vi "Crossing Balls.vi"() -> ()   [LabVIEW 2023]
uses:
  Crossing Balls.ctl
  <vilib>/numeric/Random Number (Range) U64.vi
  <vilib>/numeric/sub_Random U32.vi
panel:
  out "Combinations":i32
  out "2D Picture":picture
  in  "stop":bool
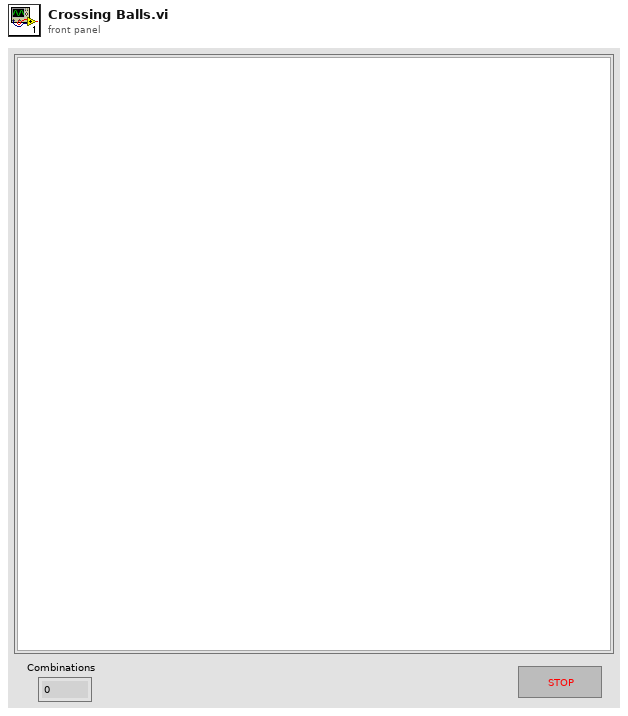
[diagram p1: front panel]
types:
  T1 = typedef "Crossing Balls.ctl" = enum16{"initialize", "InRange", "DrawPicture"}
  T2 = cluster{"horizontal":enum16{"left", "center", "right"}, "vertical":enum16{"top", "center", "bottom"}}
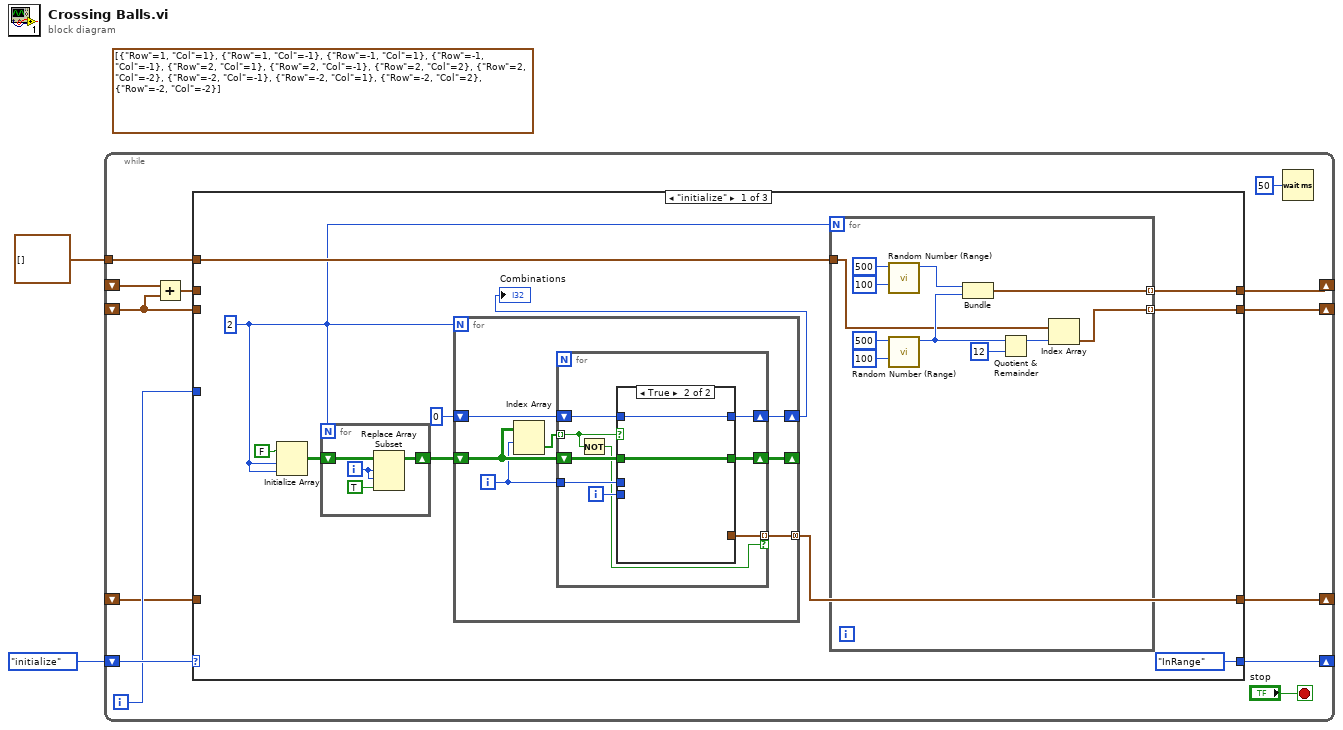
[diagram p0: block diagram]
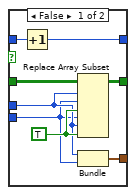
[diagram p2: hidden frame]
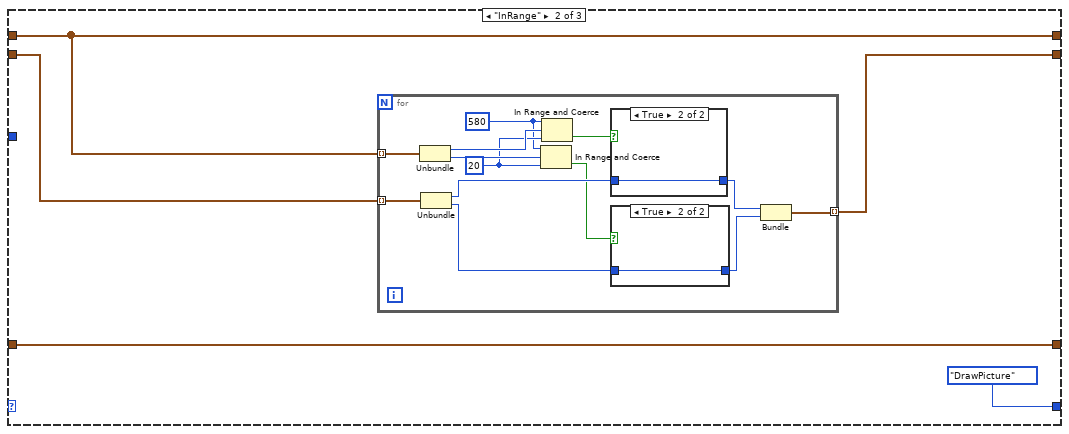
[diagram p3: hidden frame]
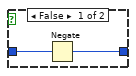
[diagram p4: hidden frame]
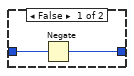
[diagram p5: hidden frame]
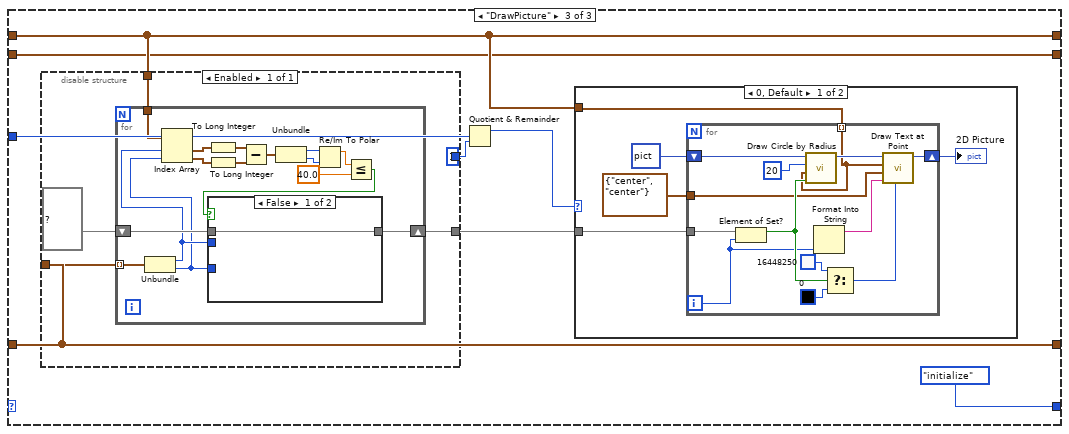
[diagram p6: hidden frame]
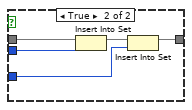
[diagram p7: hidden frame]
diagram:
  (unwired) cluster{"Row":i32, "Col":i32}[] [{"Row"=1, "Col"=1}, {"Row"=1, "Col"=-1}, {"Row"=-1, "Col"=1}, {"Row"=-1, "Col"=-1}, {"Row"=2, "Col"=1}, {"Row"=2, "Col"=-1}, {"Row"=2, "Col"=2}, {"Row"=2, "Col"=-2}, {"Row"=-2, "Col"=-1}, {"Row"=-2, "Col"=1}, {"Row"=-2, "Col"=2}, {"Row"=-2, "Col"=-2}]
  n1 = while {
    shift-right: [w12] -> _
    shift-left: Crossing_Balls."initialize" -> [w13]
    tunnel: cluster{i32, i32}[] [] -> [w10]
    shift-right: [w8] -> _
    shift-left: _ -> [w5]
    shift-right: [w9] -> _
    shift-left: _ -> [w7]
    shift-right: [w4] -> _
    shift-left: _ -> [w3]
    i -> [w11]
    stop <- "stop" stop-if-true
    n2 = Add(x=w7, y=w5) -> (x+y=w6:cluster{u64, u64}[])
    n3 = case shown="\"initialize\"" w13 {
      tunnel: w10 -> [w26 _ _]
      tunnel: [Crossing_Balls."InRange" enum16{"initialize", "InRange", "DrawPicture"}."DrawPicture" Crossing_Balls."initialize"] -> w12
      tunnel: w11 -> [_ _ w99]
      tunnel: [w25 w71 w96] -> w9
      tunnel: [w24 w69 w94] -> w8
      tunnel: w6 -> [_ w71 w96]
      tunnel: w5 -> [_ w70 w94]
      tunnel: [w17 w68 w93] -> w4
      tunnel: w3 -> [_ w68 w93]
      frame "initialize" {
        w16 = 2
        n4 = Initialize Array(FALSE, w16, w16) -> (w21:bool[][])
        n5 = for {
          N: w16 -> [_]
          shift-right: [w53] -> w20
          shift-left: w21 -> [w56]
          i -> [w55]
          n6 = Replace Array Subset(array=w56, new element=TRUE ("new element/subarray"), index (row)=w55, index (col)=w55) -> (w53:bool[][])
        }
        n7 = for {
          N: w16 -> [_]
          shift-right: [w28] -> _
          shift-left: w20 -> [w33]
          shift-right: [w29] -> w18
          shift-left: 0 -> [w30]
          tunnel: [w27] -> w17 mode=concatenating
          i -> [w31]
          n8 = Index Array(array=w33, index (row)=w31) -> (element=w32:bool[])  [unwired: 1 in]
          n9 = for {
            shift-right: [w39] -> w28
            shift-left: w33 -> [w42]
            tunnel: w32 -> [w36] mode=indexing
            tunnel: w31 -> [w41]
            shift-right: [w37] -> w29
            shift-left: w30 -> [w38]
            tunnel: [w35] -> w27 mode=indexing if=w34
            i -> [w40]
            n10 = Not(x=w36) -> (.not. x?=w34:bool)
            n11 = case shown="True" w36 {
              tunnel: w42 -> [w50 w51]
              tunnel: w41 -> [w45 _]
              tunnel: w40 -> [w44 _]
              tunnel: [w49 w51] -> w39
              tunnel: w38 -> [w47 w52]
              tunnel: [w46 w52] -> w37
              tunnel: [w43 _] -> w35
              frame False {
                w48 = TRUE
                n12 = Increment(x=w47) -> (x+1=w46:i32)
                n13 = Replace Array Subset(array=w50, new element #1=w48, index (row) #1=w45, index (col) #1=w44, new element #2=w48, index (row) #2=w44, index (col) #2=w45) -> (w49:bool[][])
                n14 = Bundle(w45, w44) -> (w43:cluster{i32, i32})  [unwired: 1 in]
              }
              frame True {
              }
            }
          }
        }
        "Combinations" <- w18
        n15 = for {
          N: w16 -> [_]
          tunnel: [w59] -> w25 mode=indexing
          tunnel: [w58] -> w24 mode=indexing
          tunnel: w26 -> [w57]
          n16 = call-poly <vilib>:"Random Number (Range).vi"("lower bound (0)"=u64 100, "upper bound (100)"=u64 500) -> ("number"=w63:u64)  [unwired: 9 in]
          n17 = call-poly <vilib>:"Random Number (Range).vi"("lower bound (0)"=u64 100, "upper bound (100)"=u64 500) -> ("number"=w62:u64)  [unwired: 9 in]
          n18 = Bundle("number"=w63, "number"=w62) -> (w59:cluster{"number":u64, "number":u64})  [unwired: 1 in]
          n19 = Quotient & Remainder(x=w62, y=u64 12) -> (x-y*floor(x/y)=w60:u64)  [unwired: 1 out]
          n20 = Index Array(array=w57, index=w60) -> (element=w58:cluster{i32, i32})
        }
      }
      frame "InRange" {
        n21 = for {
          tunnel: w71 -> [w85] mode=indexing
          tunnel: w70 -> [w84] mode=indexing
          tunnel: [w73] -> w69 mode=indexing
          w75 = u64 20 ("lower limit")
          w74 = u64 580 ("upper limit")
          n22 = Unbundle(w85) -> (w82:u64, w83:u64)
          n23 = Unbundle(w84) -> (w81:i32, w79:i32)
          n24 = In Range and Coerce(upper limit=w74, x=w83, lower limit=w75) -> (In Range?=w76:bool)  [unwired: 1 out]
          n25 = In Range and Coerce(upper limit=w74, x=w82, lower limit=w75) -> (In Range?=w77:bool)  [unwired: 1 out]
          n26 = case shown="True" w77 {
            tunnel: w81 -> [w90 w91]
            tunnel: [w89 w91] -> w80
            frame False {
              n27 = Negate(x=w90) -> (-x=w89:i32)
            }
            frame True {
            }
          }
          n28 = case shown="True" w76 {
            tunnel: w79 -> [w87 w88]
            tunnel: [w86 w88] -> w78
            frame False {
              n29 = Negate(x=w87) -> (-x=w86:i32)
            }
            frame True {
            }
          }
          n30 = Bundle(w80, w78) -> (w73:cluster{i32, i32})  [unwired: 1 in]
        }
      }
      frame "DrawPicture" {
        n31 = disable-structure shown="Enabled" {
          disable-tunnel: [w103] -> w98
          disable-tunnel: w96 -> [w102]
          disable-tunnel: w93 -> [w101]
          disable-tunnel: [1 ("y")] -> w92
          frame Enabled {
            n32 = for {
              shift-right: [w109] -> w103
              shift-left: set{i32} {} ("set") -> [w110]
              tunnel: w102 -> [w120]
              tunnel: w101 -> [w107] mode=indexing
              n33 = Unbundle(w107) -> (w106:i32, w105:i32)
              n34 = Index Array(array=w120, index #1=w106, index #2=w105) -> (element #1=w119:cluster{u64, u64}, element #2=w118:cluster{u64, u64})
              n35 = To Long Integer(number=w119) -> (32bit integer=w116:cluster{i32, i32})
              n36 = To Long Integer(number=w118) -> (32bit integer=w117:cluster{i32, i32})
              n37 = Subtract(x=w116, y=w117) -> (x-y=w115:cluster{i32, i32})
              n38 = Unbundle(w115) -> (w114:i32, w113:i32)
              n39 = Re/Im To Polar(2:w113, 3:w114) -> (1:w112:dbl)  [unwired: 1 out]
              n40 = Less Or Equal?(x=w112, y=40.0) -> (x <= y?=w108:bool)
              n41 = case shown="False" w108 {
                tunnel: w110 -> [w121 w126]
                tunnel: [w121 w124] -> w109
                tunnel: w106 -> [_ w123]
                tunnel: w105 -> [_ w122]
                frame False {
                }
                frame True {
                  n42 = Insert Into Set(10:w123, 11:w126) -> (3:w125:set{i32})  [unwired: 1 out]
                  n43 = Insert Into Set(10:w122, 11:w125) -> (3:w124:set{i32})  [unwired: 1 out]
                }
              }
            }
          }
        }
        n44 = Quotient & Remainder(x=w99, y=w92) -> (x-y*floor(x/y)=w95:i32)  [unwired: 1 out]
        n45 = case shown="0, Default" w95 {
          tunnel: w98 -> [w128 _]
          tunnel: w96 -> [w127 _]
          frame 0, Default {
            n46 = for {
              shift-right: [w141] -> w130
              shift-left: picture data[5B] ("picture") -> [w140]
              tunnel: T2 {"horizontal"=enum."center", "vertical"=enum."center"} ("alignment(left, top)") -> [w134]
              tunnel: w128 -> [w133]
              tunnel: w127 -> [w132] mode=indexing
              i -> [w139]
              n47 = Element of Set?(10:w139, 11:w133) -> (3:w143:bool)
              n48 = call <vilib>:"Draw Circle by Radius.vi"("fill?(F)"=w143, "pixel center"=w132, "radius"=i16 20, "picture"=w140) -> ("new picture"=w142:picture)  [unwired: 7 in]
              n49 = Format Into String(w139) -> (resulting string=w138:string)  [unwired: 3 in, 1 out]
              n50 = Select(t=u32 16448250 ("text color(black)"), s=w143, f=u32 0 ("text color(black)")) -> (s? t:f=w135:u32)
              n51 = call <vilib>:"Draw Text at Point.vi"("text color(black)"=w135, "text"=w138, "alignment(left, top)"=w134, "origin"=w132, "picture"=w142) -> ("new picture"=w141:picture)  [unwired: 5 in, 1 out]
            }
            "2D Picture" <- w130
          }
          frame 1 {
          }
        }
      }
    }
    n52 = Wait (ms)(milliseconds to wait=u32 50) -> ()  [unwired: 1 out]
  }
